vi "Miniquads.CalculateVoltage.vi"(1 "Miniquad Voltages":dbl[](array[numeric])) -> (15 "ChannelVoltages":dbl[](array[numeric]))   [LabVIEW 2014, in "Miniquads.lvlib"]
doc: "Calculates the channel voltages from the Miniquad voltages."
uses:
  Miniquads.lvlib
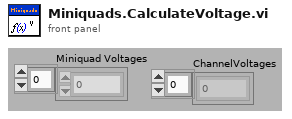
[diagram p1: front panel]
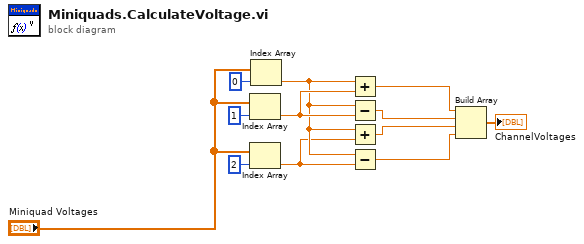
[diagram p0: block diagram]
diagram:
  n1 = Index Array(array="Miniquad Voltages", index=1 ("Index")) -> (element=w8:dbl)
  n2 = Index Array(array="Miniquad Voltages", index=2 ("Index")) -> (element=w6:dbl)
  n3 = Index Array(array="Miniquad Voltages", index=0 ("Index")) -> (element=w7:dbl)
  n4 = Add(x=w7, y=w8) -> (x+y=w5:dbl)
  n5 = Subtract(x=w7, y=w8) -> (x-y=w4:dbl)
  n6 = Add(x=w7, y=w6) -> (x+y=w3:dbl)
  n7 = Subtract(x=w7, y=w6) -> (x-y=w2:dbl)
  n8 = Build Array(w5, w4, w3, w2) -> (→"ChannelVoltages":dbl[])
